vi "relay_write.vi"(1 "on/off":bool, 2 "No.":u8=1) -> (0 "write buffer":string)   [LabVIEW 2023]
panel:
  in  "Relay COM":refnum<visa-resource-name>="COM4"
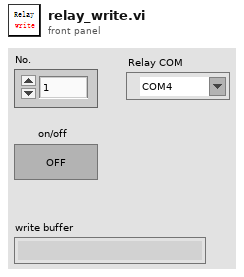
[diagram p1: front panel]
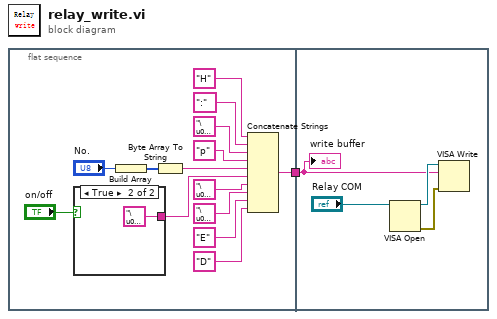
[diagram p0: block diagram]
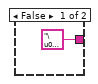
[diagram p2: hidden frame]
diagram:
  n1 = flat-sequence {
    tunnel: [w13] -> w1
    tunnel: w1 -> [w18]
    frame #0 {
      n2 = case shown="True" "on/off" {
        tunnel: ["\u0000" ("string") "\u0001" ("string")] -> w6
        frame False {
        }
        frame True {
        }
      }
      n3 = Build Array("No.") -> (w9:u8[])
      n4 = Byte Array To String(unsigned byte array=w9) -> (string=w8:string)
      n5 = Concatenate Strings("H" ("string"), ":" ("string"), "\u0001" ("string"), "p" ("string"), w8, w6, "\u0000" ("string"), "\u0000" ("string"), "E" ("string"), "D" ("string")) -> (w13:string)
    }
    frame #1 {
      n6 = VISA Open(VISA resource name="Relay COM") -> (VISA resource name=w21:refnum<visa-resource-name>, error out=w19:errorcluster)  [unwired: 4 in]
      n7 = VISA Write(VISA resource name=w21, write buffer=w18, error in (no error)=w19) -> ()  [unwired: 3 out]
      "write buffer" <- w18
    }
  }
